vi "save_direction.vi"(9 "Path":path, 10 "Direction":string) -> ()   [LabVIEW 2012]
uses:
  Global_var.vi
panel:
  out "cur_path":path
  out "error out":errorcluster
  out "Center":dbl[](array[numeric]) format="%#_3g"
  in  "No":bool
  in  "Yes":bool
  # "The program will now save the extreme direction:        degree for our current patient. \n\nPress YES to continue, or NO to decline."
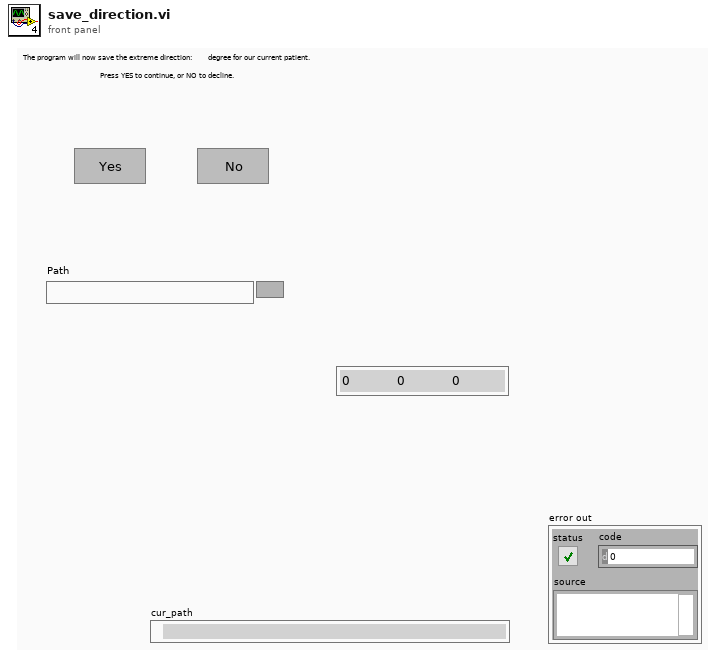
[diagram p1: front panel]
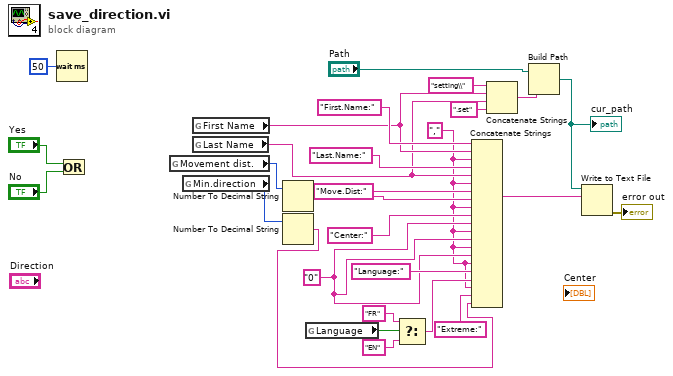
[diagram p0: block diagram]
diagram:
  w10 = "0"
  w4 = ","
  n1 = Wait (ms)(milliseconds to wait=u32 50) -> ()  [unwired: 1 out]
  n2 = Or(x="Yes", y="No") -> ()  [unwired: 1 out]
  n3 = global read "Global_var.vi" "Movement dist."() -> (w7:u8)
  n4 = global read "Global_var.vi" "Min.direction"() -> (w6:i8)
  n5 = global read "Global_var.vi" "First Name"() -> (w9:string)
  n6 = global read "Global_var.vi" "Last Name"() -> (w8:string)
  n7 = Number To Decimal String(number=w7) -> (decimal integer string=w19:string)  [unwired: 1 in]
  n8 = Number To Decimal String(number=w6) -> (decimal integer string=w2:string)  [unwired: 1 in]
  n9 = global read "Global_var.vi" "Language"() -> (w5:bool)
  n10 = Select(t="FR", s=w5, f="EN") -> (s? t:f=w25:string)
  n11 = Concatenate Strings("First.Name:", w9, w4, "Last.Name:", w8, w4, "Move.Dist:", w19, w4, "Center:", w10, w4, w10, w4, w10, w4, "Language:", w25, w4, "Extreme:", w2) -> (w14:string)
  n12 = Concatenate Strings("setting\\" ("string"), w9, w8, ".set" ("string")) -> (w21:string)
  n13 = Build Path(base path="Path", name or relative path=w21) -> (appended path=w20:path)
  "cur_path" <- w20
  n14 = Write to Text File(file (use dialog)=w20, text=w14) -> (error out=→"error out":errorcluster)  [unwired: 2 in, 2 out]
